vi "Read Specific DAC Cfg.vi"(8 "error in":errorcluster, 10 "Default Config File Refnum":T1, 11 "DAC in":refnum<class "DAC.lvclass">) -> (0 "error out":errorcluster, 1 "Correct file?":bool, 2 "refnum out":T1, 3 "DAC out":refnum<class "DAC.lvclass">)   [LabVIEW 2019, in "DAC.lvlib" / "DAC.lvclass"]
uses:
  DAC.lvclass
  <vilib>/Utility/config.llb/Config Data RefNum.ctl
  DAC.lvclass/DAC.ctl
  <vilib>/Utility/config.llb/Read Key (String).vi
  <vilib>/Utility/config.llb/Read Key (Double).vi
  <vilib>/Utility/config.llb/NI_LVConfig.lvlib
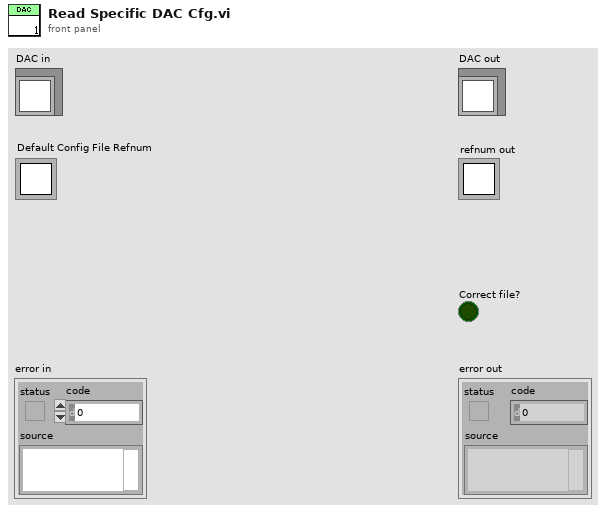
[diagram p1: front panel]
types:
  T1 = typedef "NI_LVConfig.lvlib/Config Data RefNum.ctl" = refnum<k1>
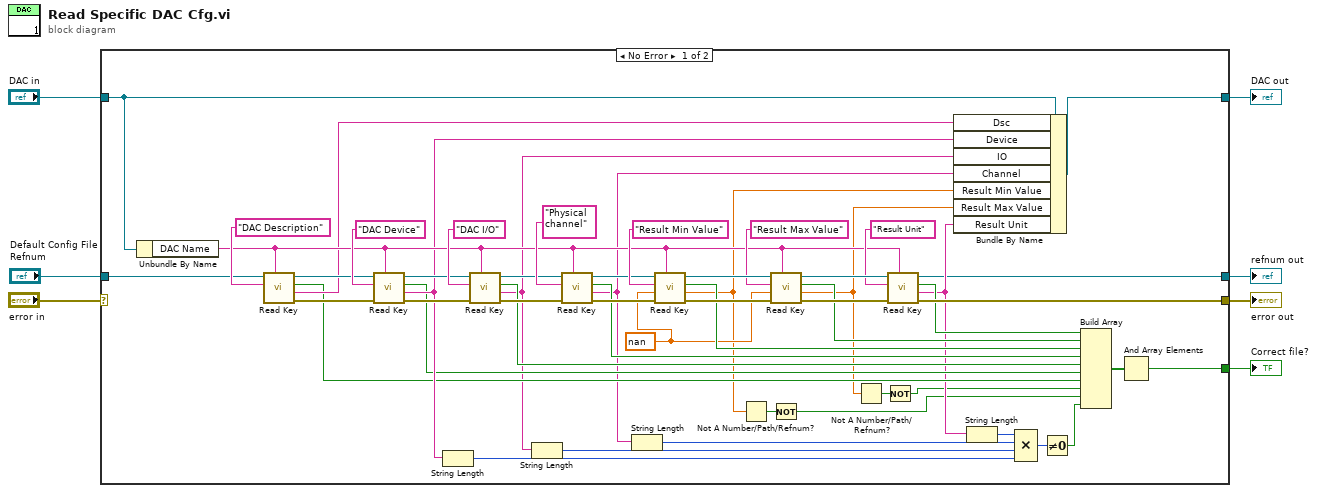
[diagram p0: block diagram]
diagram:
  n1 = case shown="No Error" "error in" {
    selector: "error in" -> [_ w62]
    tunnel: [w35 w62] -> w6
    tunnel: [w37 w61] -> w4
    tunnel: "DAC in" -> [w40 w61]
    tunnel: "Default Config File Refnum" -> [w38 w60]
    tunnel: [w9 _] -> w2
    tunnel: [w8 w60] -> w1
    frame No Error {
      w19 = nan
      n2 = Unbundle By Name(w40) -> ("DAC Name"=w39:string)
      n3 = call-poly <vilib>:"Read Key.vi"("section"=w39, "key"="DAC Description", "refnum"=w38) -> ("error out"=w43:errorcluster, "value"=w36:string, "found?"=w33:bool, "refnum out"=w42:T1)  [unwired: 5 in]
      n4 = call-poly <vilib>:"Read Key.vi"("section"=w39, "error in (no error)"=w43, "key"="DAC Device", "refnum"=w42) -> ("error out"=w44:errorcluster, "value"=w34:string, "found?"=w32:bool, "refnum out"=w41:T1)  [unwired: 4 in]
      n5 = String Length(string=w34) -> (length=w20:i32)
      n6 = call-poly <vilib>:"Read Key.vi"("section"=w39, "error in (no error)"=w44, "key"="DAC I/O", "refnum"=w41) -> ("error out"=w48:errorcluster, "value"=w26:string, "found?"=w31:bool, "refnum out"=w49:T1)  [unwired: 4 in]
      n7 = String Length(string=w26) -> (length=w21:i32)
      n8 = call-poly <vilib>:"Read Key.vi"("section"=w39, "error in (no error)"=w48, "key"="Physical channel", "refnum"=w49) -> ("error out"=w46:errorcluster, "value"=w25:string, "found?"=w30:bool, "refnum out"=w47:T1)  [unwired: 4 in]
      n9 = String Length(string=w25) -> (length=w22:i32)
      n10 = call-poly <vilib>:"Read Key.vi"("section"=w39, "error in (no error)"=w46, "default value"=w19, "key"="Result Min Value", "refnum"=w47) -> ("error out"=w56:errorcluster, "value"=w18:dbl, "found?"=w29:bool, "refnum out"=w58:T1)  [unwired: 3 in]
      n11 = Not A Number/Path/Refnum?(number/path/refnum=w18) -> (NaN/Path/Refnum?=w16:bool)
      n12 = call-poly <vilib>:"Read Key.vi"("section"=w39, "error in (no error)"=w56, "default value"=w19, "key"="Result Max Value", "refnum"=w58) -> ("error out"=w55:errorcluster, "value"=w17:dbl, "found?"=w28:bool, "refnum out"=w57:T1)  [unwired: 3 in]
      n13 = Not(x=w16) -> (.not. x?=w13:bool)
      n14 = Not A Number/Path/Refnum?(number/path/refnum=w17) -> (NaN/Path/Refnum?=w15:bool)
      n15 = Not(x=w15) -> (.not. x?=w14:bool)
      n16 = call-poly <vilib>:"Read Key.vi"("section"=w39, "error in (no error)"=w55, "key"="Result Unit", "refnum"=w57) -> ("error out"=w35:errorcluster, "value"=w24:string, "found?"=w27:bool, "refnum out"=w8:T1)  [unwired: 4 in]
      n17 = Bundle By Name(cluster=w40, "Dsc"=w36, "Device"=w34, "IO"=w26, "Channel"=w25, "Result Min Value"=w18, "Result Max Value"=w17, "Result Unit"=w24) -> (w37:refnum<class "DAC.lvclass">)
      n18 = String Length(string=w24) -> (length=w23:i32)
      n19 = Compound Arithmetic op=MULTIPLY(w23, w22, w21, w20) -> (w12:i32)
      n20 = Not Equal To 0?(x=w12) -> (x != 0?=w11:bool)
      n21 = Build Array(w27, w28, w29, w30, w31, w32, w33, w14, w13, w11) -> (w10:bool[])
      n22 = And Array Elements(Boolean array=w10) -> (logical AND=w9:bool)
    }
    frame Error {
    }
  }
  "error out" <- w6
  "DAC out" <- w4
  "Correct file?" <- w2
  "refnum out" <- w1
